vi "HtmlJsTemplate.vi"(10 "js":T1, 11 "HTML":T2) -> (2 "js out":string, 3 "HTML out":string)   [LabVIEW 2014, in "WebFrontPanel.lvclass"]
uses:
  WebFrontPanel.lvclass
  Controls/HTMLTemplateFill.ctl
  Controls/JSTemplateFill.ctl
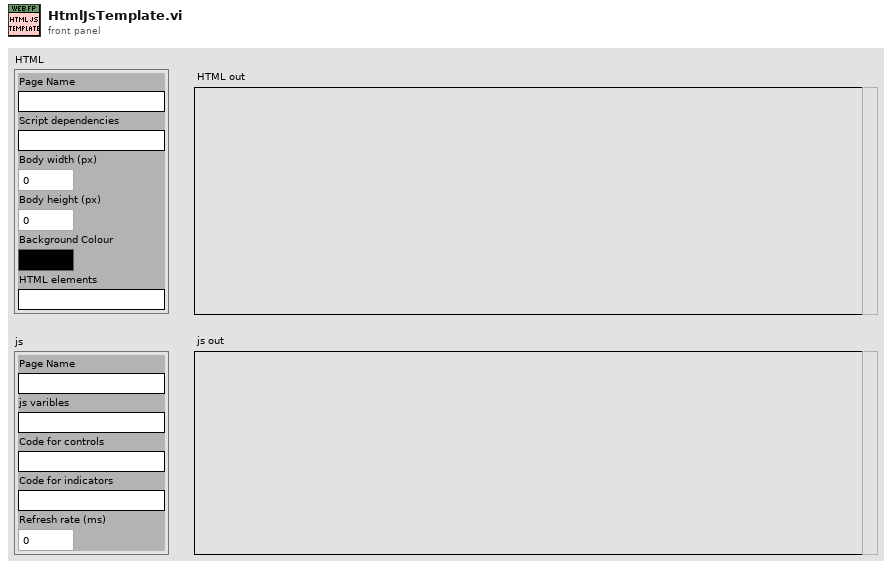
[diagram p1: front panel]
types:
  T1 = typedef "WebFrontPanel.lvclass/JSTemplateFill.ctl" = cluster{"Page Name":string, "js varibles":string, "Code for controls":string, "Code for indicators":string, "Refresh rate (ms)":i32}
  T2 = typedef "WebFrontPanel.lvclass/HTMLTemplateFill.ctl" = cluster{"Page Name":string, "Script dependencies":string, "Body width (px)":i32, "Body height (px)":i32, "Background Colour":u32, "HTML elements":string}
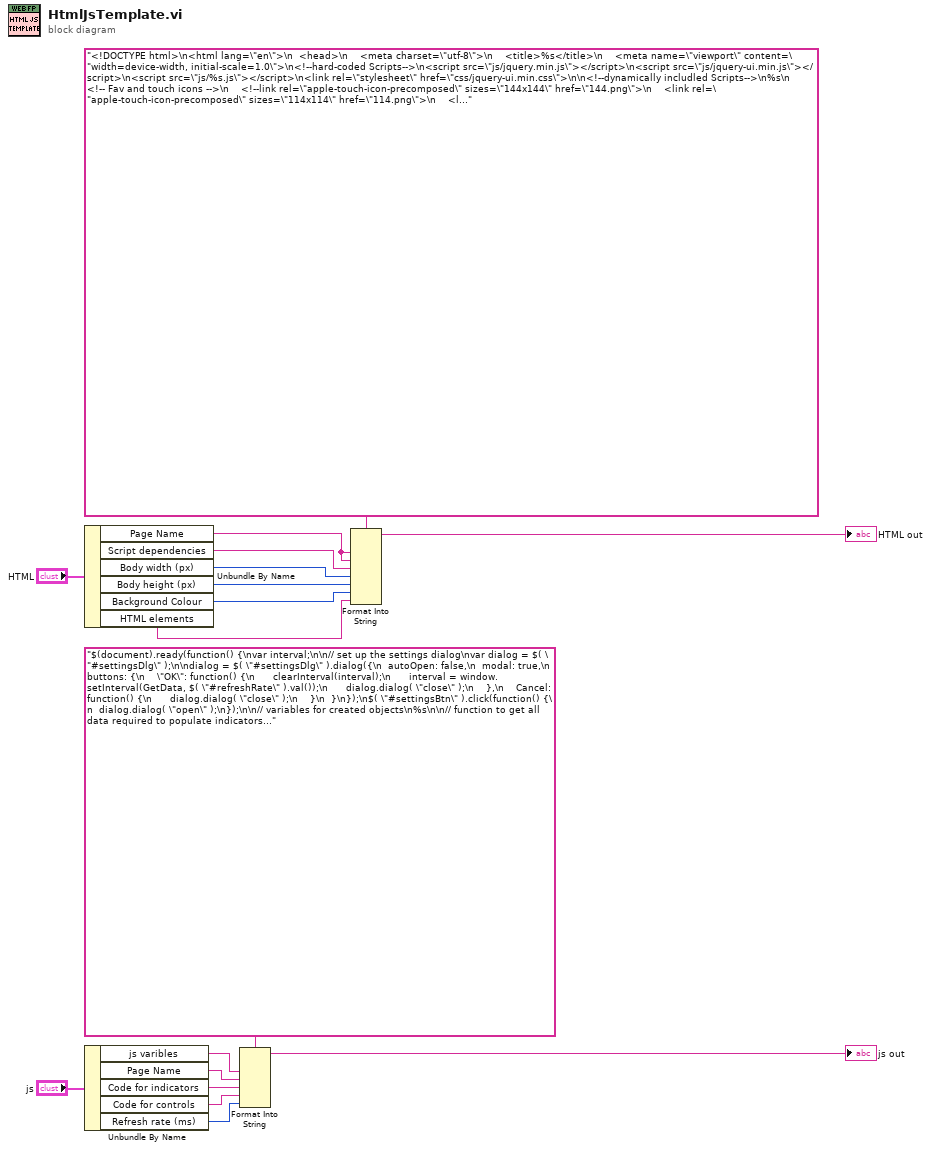
[diagram p0: block diagram]
diagram:
  n1 = Unbundle By Name("HTML") -> ("Page Name"=w14:string, "Script dependencies"=w13:string, "Body width (px)"=w12:i32, "Body height (px)"=w11:i32, "Background Colour"=w1:u32, "HTML elements"=w2:string)
  n2 = Unbundle By Name("js") -> ("js varibles"=w7:string, "Page Name"=w6:string, "Code for indicators"=w5:string, "Code for controls"=w4:string, "Refresh rate (ms)"=w3:i32)
  n3 = Format Into String(format string="$(document).ready(function() {\nvar interval;\n\n// set up the settings dialog\nvar dialog = $( \"#settingsDlg\" );\n\ndialog = $( \"#settingsDlg\" ).dialog({\n  autoOpen: false,\n  modal: true,\n  buttons: {\n    \"OK\": function() {\n      clearInterval(interval);\n      interval = window.setInterval(GetData, $( \"#refreshRate\" ).val());\n      dialog.dialog( \"close\" );\n    },\n    Cancel: function() {\n      dialog.dialog( \"close\" );\n    }\n  }\n});\n$( \"#settingsBtn\" ).click(function() {\n  dialog.dialog( \"open\" );\n});\n\n// variables for created objects\n%s\n\n// function to get all data required to populate indicators\nfunction GetData(){\n\t$.get(\"GetData?Page=%s\", \n\t\tfunction(res){\n// object specific code to manipulate variables defined above\n%s\n\t\t},\n\t\t\"json\");\n};\n\n// Additional functions for controls\n%s\n\n// set data refresh rate\ninterval = window.setInterval(GetData, %d);\n\n});", w7, w6, w5, w4, w3) -> (resulting string=→"js out":string)  [unwired: 2 in, 1 out]
  n4 = Format Into String(format string="<!DOCTYPE html>\n<html lang=\"en\">\n  <head>\n    <meta charset=\"utf-8\">\n    <title>%s</title>\n    <meta name=\"viewport\" content=\"width=device-width, initial-scale=1.0\">\n<!--hard-coded Scripts-->\n<script src=\"js/jquery.min.js\"></script>\n<script src=\"js/jquery-ui.min.js\"></script>\n<script src=\"js/%s.js\"></script>\n<link rel=\"stylesheet\" href=\"css/jquery-ui.min.css\">\n\n<!--dynamically includled Scripts-->\n%s\n    <!-- Fav and touch icons -->\n    <!--link rel=\"apple-touch-icon-precomposed\" sizes=\"144x144\" href=\"144.png\">\n    <link rel=\"apple-touch-icon-precomposed\" sizes=\"114x114\" href=\"114.png\">\n    <link rel=\"apple-touch-icon-precomposed\" sizes=\"72x72\" href=\"72.png\">\n    <link rel=\"apple-touch-icon-precomposed\" href=\"57.png\"-->\n    <link rel=\"shortcut icon\" href=\"favicon.ico\">\n  </head>\n\n  <body style=\"position: fixed; width: %dpx; height: %dpx;border-radius: 5px; border: 1px solid #000000; background-color: #%x;\">\n%s\n  <div id=\"settingsDlg\" title=\"Settings\"><form><fieldset>\n    <label>Refresh rate (ms):</label>\n    <input type=\"text\" name=\"refreshRate\" id=\"refreshRate\" value=\"250\" class=\"text ui-widget-content ui-corner-all\"></fieldset></form>\n  </div>\n  <img id=\"settingsBtn\" style=\"position: fixed; bottom: 0px; right: 0px;\" src=\"img/cog.png\" title=\"Settings\">\n</body>\n</html>", w14, w14, w13, w12, w11, w1, w2) -> (resulting string=→"HTML out":string)  [unwired: 2 in, 1 out]
